vi "increment-file-name.vi"(11 "name or relative path":string) -> (3 "concatenated string":string)   [LabVIEW 2013]
uses:
  <vilib>/regexp/Match Regular Expression.xnode
panel:
  out "whole match":string
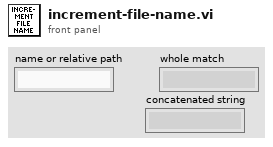
[diagram p1: front panel]
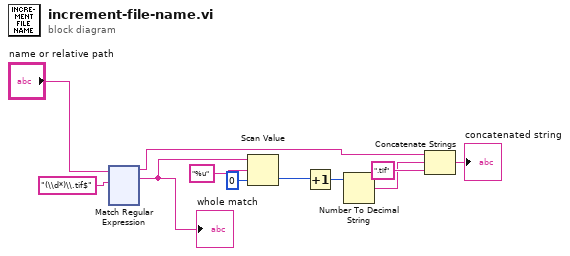
[diagram p0: block diagram]
diagram:
  n1 = xnode "Match Regular Expression"("input string"="name or relative path", "regular expression"="(\\d*)\\.tif$") -> ("before match"=w11:string, "whole match"=w10:string)  [unwired: 4 in, 3 out]
  "whole match" <- w10
  n2 = Scan Value(string=w10, format string="%u", default (0 dbl)=u32 0) -> (value=w5:u32)  [unwired: 1 out]
  n3 = Increment(x=w5) -> (x+1=w6:u32)
  n4 = Number To Decimal String(number=w6) -> (decimal integer string=w7:string)  [unwired: 1 in]
  n5 = Concatenate Strings(w11, w7, ".tif" ("string")) -> (→"concatenated string":string)
